vi "Party Time Drive Too - Joysticks.vi"(11 "Controller Values":T1) -> (2 "Right Setpoint":dbl, 3 "Left Setpoint":dbl)   [LabVIEW 2018]
uses:
  Controller Values.ctl
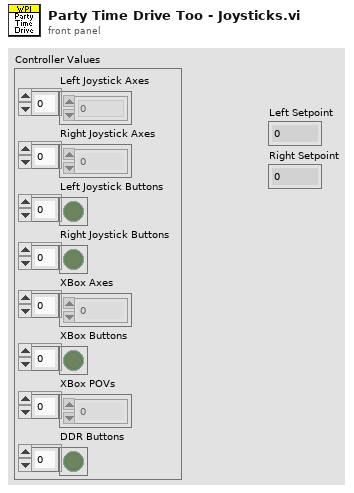
[diagram p1: front panel]
types:
  T1 = typedef "Controller Values.ctl" = cluster{"Left Joystick Axes ":dbl[], "Right Joystick Axes":dbl[], "Left Joystick Buttons":bool[], "Right Joystick Buttons":bool[], "XBox Axes":dbl[], "XBox Buttons":bool[], "XBox POVs":i16[], "DDR Buttons":bool[]}
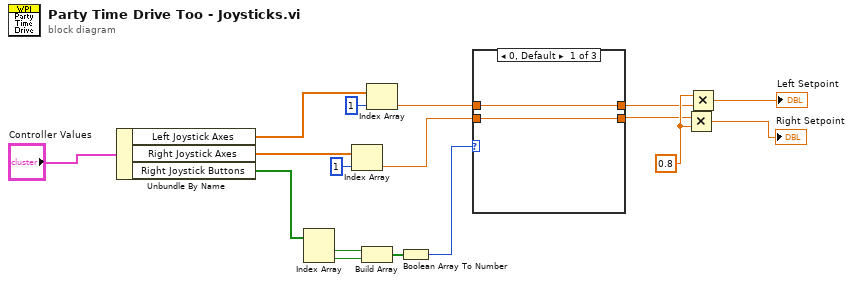
[diagram p0: block diagram]
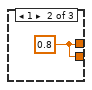
[diagram p2: hidden frame]
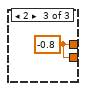
[diagram p3: hidden frame]
diagram:
  w15 = 0.8 ("y")
  n1 = Unbundle By Name("Controller Values") -> ("Left Joystick Axes"=w9:dbl[], "Right Joystick Axes"=w5:dbl[], "Right Joystick Buttons"=w6:bool[])
  n2 = Index Array(array=w6) -> (element #1=w1:bool, element #2=w2:bool)  [unwired: 2 in]
  n3 = Index Array(array=w5, index=1) -> (element=w3:dbl)
  n4 = Build Array(w1, w2) -> (w8:bool[])
  n5 = Index Array(array=w9, index=1) -> (element=w16:dbl)
  n6 = Boolean Array To Number(Boolean array=w8) -> (number=w7:u32)
  n7 = case shown="0, Default" w7 {
    tunnel: w16 -> [w19 _ _]
    tunnel: [w19 w20 w21] -> w13
    tunnel: w3 -> [w18 _ _]
    tunnel: [w18 w20 w21] -> w12
    frame 0, Default {
    }
    frame 1 {
      w20 = 0.8 ("upper limit")
    }
    frame 2 {
      w21 = -0.8 ("upper limit")
    }
  }
  n8 = Multiply(x=w12, y=w15) -> (x*y=→"Right Setpoint":dbl)
  n9 = Multiply(x=w15, y=w13) -> (x*y=→"Left Setpoint":dbl)
